vi "Move to Column.vi"(11 "Data In":T1) -> (3 "Data Out":T1)   [LabVIEW 2020]
uses:
  Data.ctl
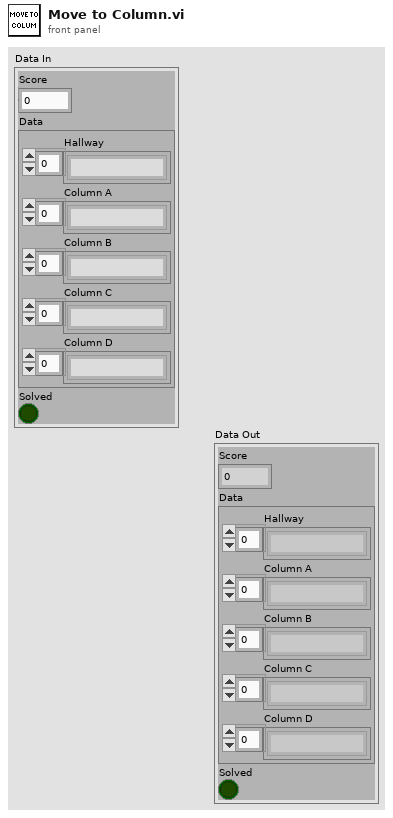
[diagram p1: front panel]
types:
  T1 = typedef "Data.ctl" = cluster{"Score":i64, "Data":cluster{"Hallway":string[], "Column A":string[], "Column B":string[], "Column C":string[], "Column D":string[]}, "Solved":bool}
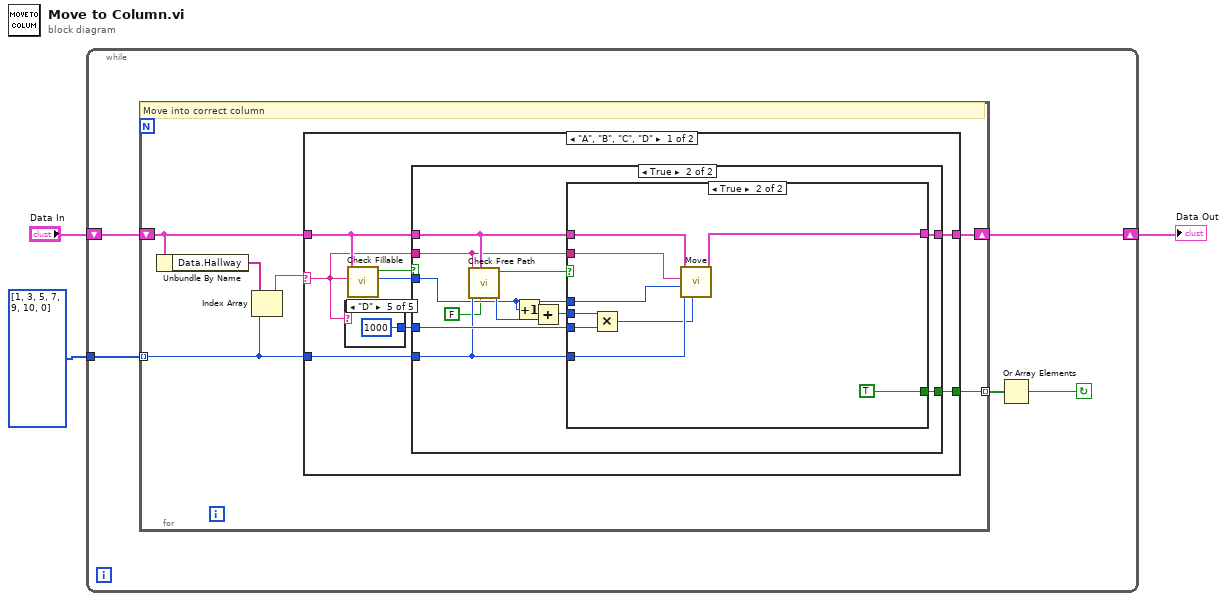
[diagram p0: block diagram]
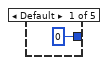
[diagram p2: hidden frame]
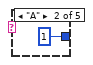
[diagram p3: hidden frame]
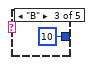
[diagram p4: hidden frame]
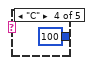
[diagram p5: hidden frame]
diagram:
  n1 = while {
    tunnel: i32[] [1, 3, 5, 7, 9, 10, 0] ("indices") -> [w7]
    shift-right: [w8] -> w2
    shift-left: "Data In" -> [w5]
    stop <- w4 continue-if-true
    n2 = for {
      tunnel: w7 -> [w14] mode=indexing
      shift-right: [w11] -> w8
      shift-left: w5 -> [w9]
      tunnel: [w10] -> w6 mode=indexing
      # "Move into correct column"
      n3 = Unbundle By Name(w9) -> ("Data.Hallway"=w12:string[])
      n4 = Index Array(array=w12, index=w14) -> (element=w13:string)
      n5 = case shown="\"A\", \"B\", \"C\", \"D\"" w13 {
        selector: w13 -> [w18 _]
        tunnel: w9 -> [w21 w51]
        tunnel: w14 -> [w19 _]
        tunnel: [w16 w51] -> w11
        tunnel: [w15 _] -> w10
        frame "A", "B", "C", "D" {
          n6 = case shown="\"D\"" w18 {
            tunnel: [i64 0 i64 1 i64 10 i64 100 i64 1000] -> w17
            frame Default {
            }
            frame "A" {
            }
            frame "B" {
            }
            frame "C" {
            }
            frame "D" {
            }
          }
          n7 = call "Check Fillable.vi"("Column"=w18, "Data In"=w21) -> ("Index"=w20:i32, "Fillable"=w22:bool)  [unwired: 8 in]
          n8 = case shown="True" w22 {
            tunnel: w21 -> [w28 w37]
            tunnel: w20 -> [_ w34]
            tunnel: w18 -> [_ w32]
            tunnel: w19 -> [_ w36]
            tunnel: w17 -> [_ w38]
            tunnel: [w28 w30] -> w16
            tunnel: [_ w29] -> w15
            frame False {
            }
            frame True {
              n9 = call "Check Free Path.vi"("To Hallway"=FALSE, "Data In"=w37, "Hallway Index"=w36, "Column"=w32) -> ("Length"=w39:i32, "Free Path?"=w40:bool)  [unwired: 6 in]
              n10 = Increment(x=w34) -> (x+1=w33:i32)
              n11 = Add(x=w33, y=w39) -> (x+y=w35:i32)
              n12 = case shown="True" w40 {
                tunnel: w35 -> [_ w49]
                tunnel: w38 -> [_ w50]
                tunnel: w37 -> [w41 w48]
                tunnel: w32 -> [_ w47]
                tunnel: w34 -> [_ w46]
                tunnel: w36 -> [_ w45]
                tunnel: [w41 w42] -> w30
                tunnel: [_ TRUE] -> w29
                frame False {
                }
                frame True {
                  n13 = Multiply(x=w49, y=w50) -> (x*y=w44:i64)
                  n14 = call "Move.vi"("Cost"=w44, "Hallway Index"=w45, "Column Index"=w46, "Column"=w47, "Data In"=w48) -> ("Data Out"=w42:T1)  [unwired: 6 in]
                }
              }
            }
          }
        }
        frame ".", Default {
        }
      }
    }
    n15 = Or Array Elements(Boolean array=w6) -> (logical OR=w4:bool)
  }
  "Data Out" <- w2
